vi "Go To Announcing.vi"(8 "error in (no error)":errorcluster, 11 "Connect Command in":refnum<class "Connect Command.lvclass">) -> (0 "error out":errorcluster, 3 "State out":refnum<class "State Actor.lvclass">)   [LabVIEW 2013, in "Receiver.lvlib" / "Receiver Commands Using Processor.lvlib" / "Connect Command.lvlib" / "Connect Command.lvclass"]
uses:
  Connect Command.lvclass
  <vilib>/ni/Actors/State Actor/State Actor/State Actor.lvclass
  Annoucing/Announcing.lvclass
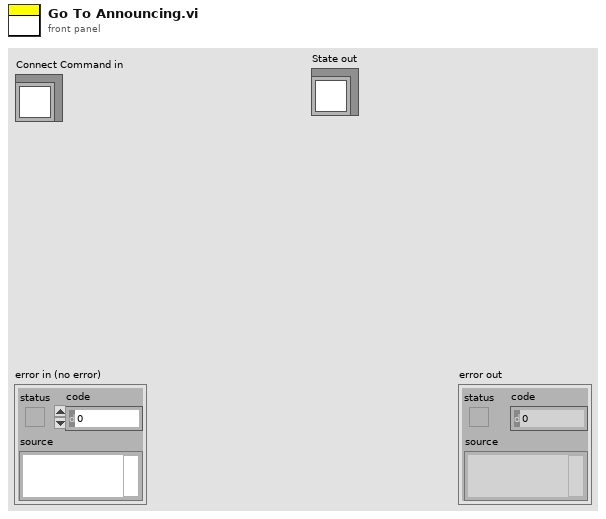
[diagram p1: front panel]
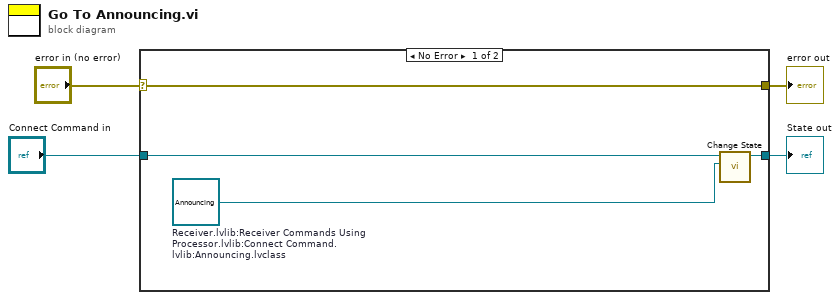
[diagram p0: block diagram]
diagram:
  n1 = case shown="No Error" "error in (no error)" {
    selector: "error in (no error)" -> [w8 w10]
    tunnel: [w8 w10] -> w3
    tunnel: [w7 w9] -> w1
    tunnel: "Connect Command in" -> [w5 w9]
    frame No Error {
      w6 = refnum<class "Announcing.lvclass"> refnum  # Receiver.lvlib:Receiver Commands Using Processor.lvlib:Connect Command.lvlib:Announcing.lvclass
      n2 = call <vilib>:"Change State.vi"("New State in"=w6, "State in"=w5) -> ("State out"=w7:refnum<class "State Actor.lvclass">)  [unwired: 8 in, 1 out]
    }
    frame Error {
    }
  }
  "error out" <- w3
  "State out" <- w1
